vi "tui_ClientSrv Remote File Manager.vi"() -> ()   [LabVIEW 2012]
doc: "Allows management of resource files on the connected server. This makes it feasible to deploy the server in a secure manner while still being able to do some basic maintenance over the network.\n\nNormally, managing files remotely requires you to open a network share. By instead limiting the server's network services to the VI-server protocol, the server becomes less vulnerable. Because all communication goes through one port, it is easy to set up an isolated subnet with forwarding of its VI-server port via an intranet gateway (e.g. using xinetd under linux). That way, the server is accessible from the intranet without being part of it. This is desirable from a security point of view since measurement machines tend to be Windows machines (because of driver support) that must keep on running and thus cannot keep up with the latest security fixes. Such machines should be isolated from the intranet. Indeed, for mission-critical tasks such isolation should be a precondition to deployment no matter how up-to-date the security fixes."
uses:
  served/ClientSrv Server File Manipulation_srv.ctl
  typedefs/t_ClientSrv Remote File Manager States.ctl
  library/typedefs/t_Library Session Methods.ctl
  typedefs/t_ClientSrv Tree Controller Methods.ctl
  typedefs/t_ClientSrv Access Levels.ctl
  typedefs/t_ClientSrv Server File Manipulation Methods.ctl
  library/glb_Library Configuration Globals.vi
panel:
  in  "local start path":path
  in  "remote start path":path
  in  "refresh remote":bool
  in  "delete remote":bool
  in  "rename remote":bool
  in  "mkdir remote":bool
  in  "new remote":bool
  in  "remote tree":string(tree)
  in  "local tree":string(tree)
  in  "refresh local":bool
  in  "delete local":bool
  in  "rename local":bool
  in  "mkdir local":bool
  in  "new local":bool
  out "file manipulation":T1
  in  "pattern":string(combo)
  in  "download":bool
  in  "upload":bool
  in  "exit":bool
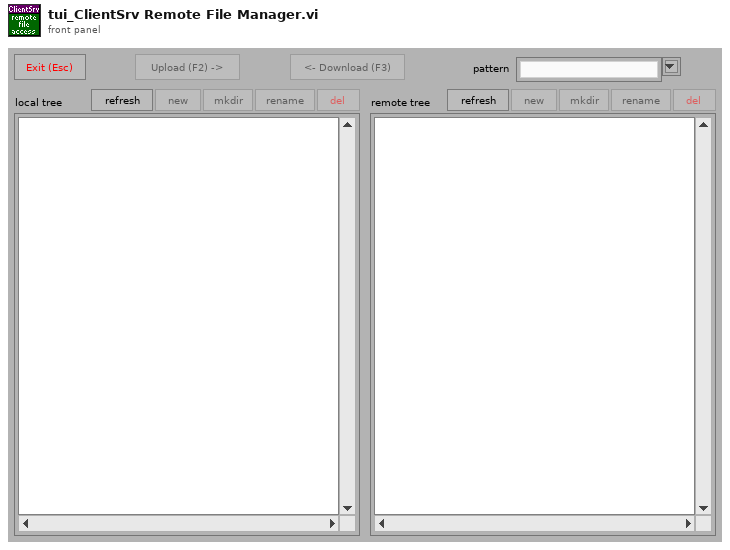
[diagram p1: front panel]
types:
  T1 = typedef "ClientSrv Server File Manipulation_srv.ctl" = refnum<vi>
  T2 = typedef "t_ClientSrv Remote File Manager States.ctl" = enum16{"empty queue", "initialize", "delayed update", "resize", "update trees", "ablement", "cleanup", "stop"}
  T3 = typedef "t_Library Session Methods.ctl" = enum16{"run", "get arg", "set arg", "delist", "cleanup?", "start session", "stop session", "list empty?"}
  T4 = typedef "t_ClientSrv Tree Controller Methods.ctl" = enum16{"do nothing", "initialize", "open item", "close item", "refresh"}
  T5 = typedef "t_ClientSrv Server File Manipulation Methods.ctl" = enum16{"close", "list", "open", "new", "read", "write", "newdir", "info", "rename", "delete"}
  T6 = typedef "t_ClientSrv Access Levels.ctl" = enum16{"observer", "operator", "local"}
  T7 = typedef "eventvkey.ctl" = enum16{"ASCII", "Enter", "Return", "Shift", "Ctrl", "Alt", "Cmd", "Opt", "Caps", "NumLock", "Clear", "Break", "Up", "Down", "Left", "Right", "Insert", "Delete", "Home", "End", "PageUp", "PageDown", "Escape", "Help", "Pause", "ScrollLock", "F1", "F2", "F3", "F4", "F5", "F6", "F7", "F8", "F9", "F10", "F11", "F12", "F13", "F14", "F15", "F16", "F17", "F18", "F19", "F20", "F21", "F22", "F23", "F24", "Play", "VolumeUp", "VolumeDown", "Mute", "Two Byte Char"}
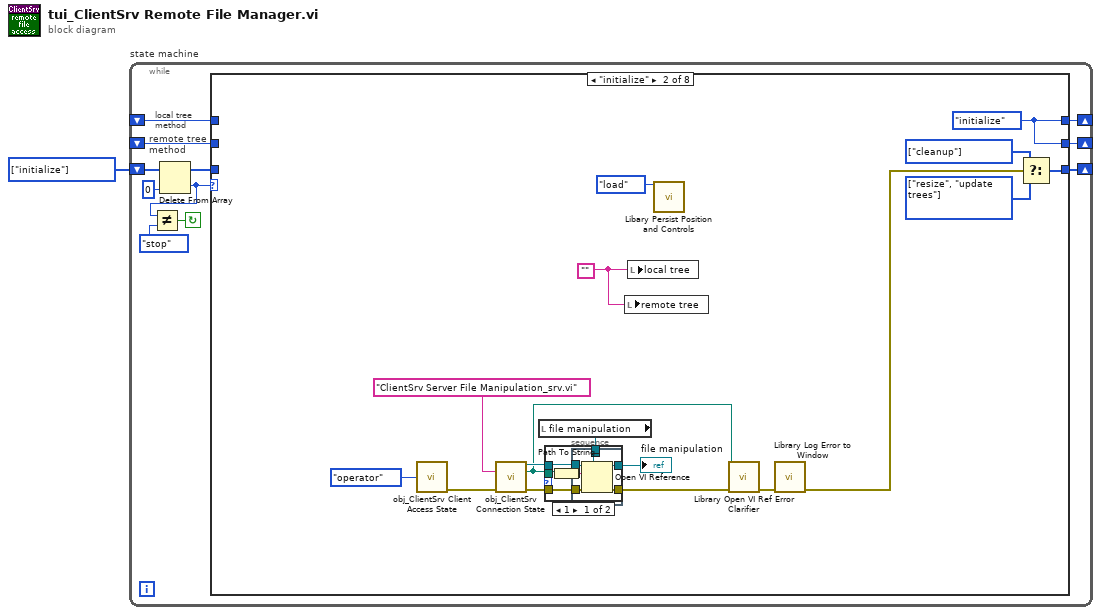
[diagram p0: block diagram]
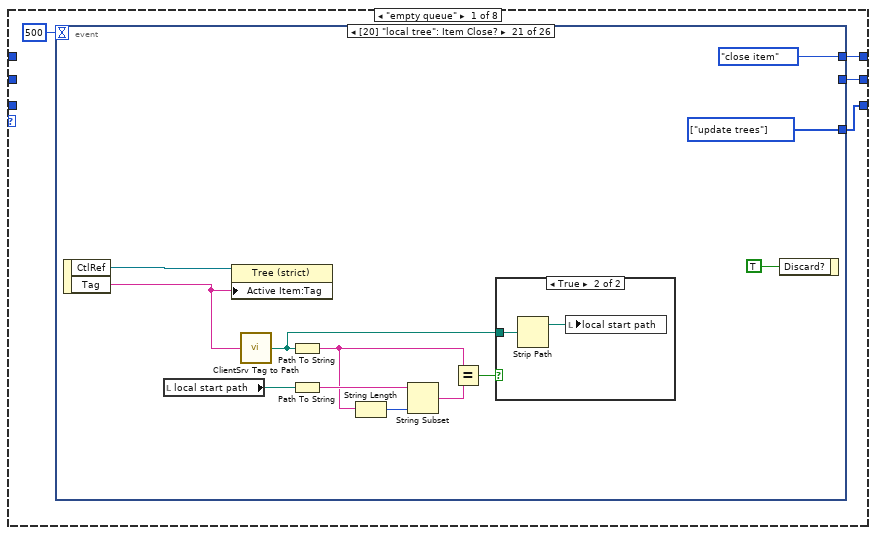
[diagram p2: hidden frame]
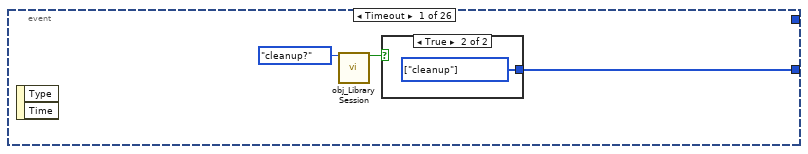
[diagram p3: hidden frame]
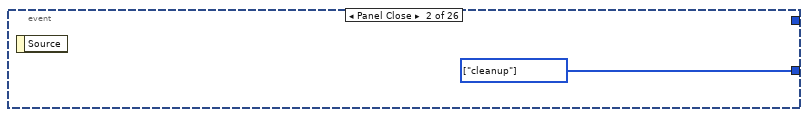
[diagram p5: hidden frame]
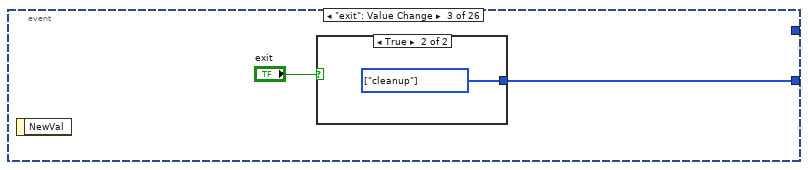
[diagram p6: hidden frame]
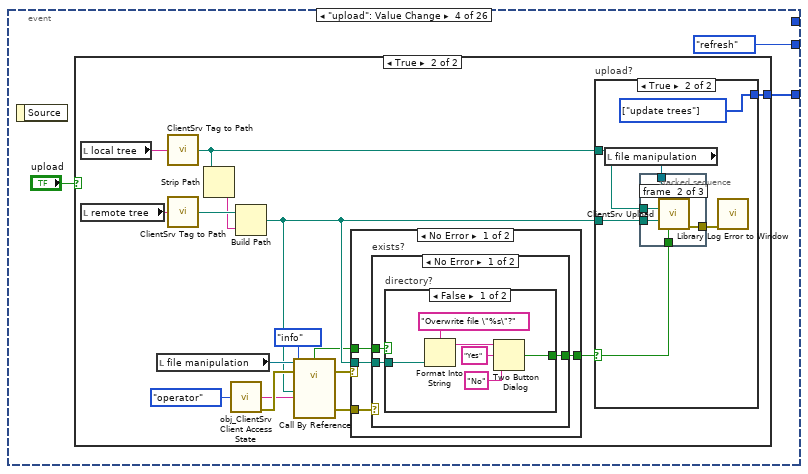
[diagram p8: hidden frame]
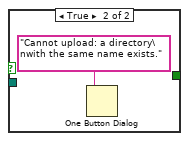
[diagram p10: hidden frame]
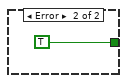
[diagram p11: hidden frame]
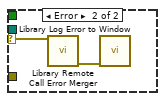
[diagram p12: hidden frame]
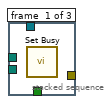
[diagram p14: hidden frame]
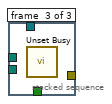
[diagram p15: hidden frame]
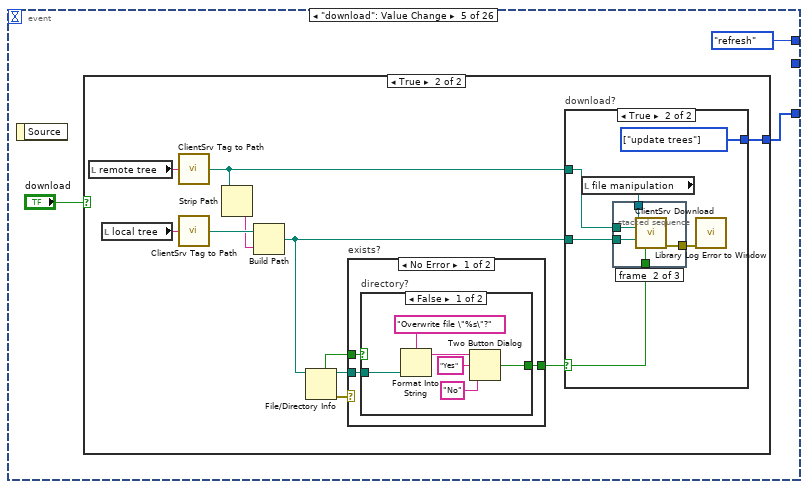
[diagram p16: hidden frame]
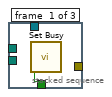
[diagram p19: hidden frame]
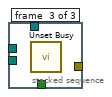
[diagram p20: hidden frame]
diagram:
  w1 = T2[] [enum."initialize"] items=["empty queue", "initialize", "delayed update", "resize", "update trees", "ablement", "cleanup", "stop"]
  n1 = while "state machine" {
    shift-right: [w12] -> _
    shift-left: w1 -> [w5]
    shift-right: [w9] -> _
    shift-left: _ -> [w11]
    shift-right: [w8] -> _
    shift-left: _ -> [w10]
    stop <- w4 continue-if-true
    # "remote tree\nmethod"
    # "local tree\nmethod"
    n2 = Delete From Array(array=w5, index=0) -> (deleted portion=w2:T2, array with subset deleted=w6:T2[])  [unwired: 1 in]
    n3 = Not Equal?(x=w2, y=t_ClientSrv_Remote_File_Manager_States."stop" ("method")) -> (x != y?=w4:bool)
    n4 = case shown="\"initialize\"" w2 {
      tunnel: [w13 w384 w412 w417 w439 w526 w611 w616] -> w12
      tunnel: w6 -> [_ _ w411 w418 w439 w526 _ w616]
      tunnel: w11 -> [_ _ w415 w421 w438 w511 w604 w615]
      tunnel: w10 -> [_ _ w414 w419 w437 w510 w603 w614]
      tunnel: [w15 w388 w415 _ w438 w511 w604 w615] -> w9
      tunnel: [w14 w388 w414 _ w437 w510 w603 w614] -> w8
      frame "empty queue" {
        n5 = event shown="[20] \"local tree\": Item Close?" {
          selector: _ -> [_ _ _ _ _ _ _ _ _ _ _ _ _ _ _ _ _ _ _ _ _ _ _ _ _ _]
          dyn-events: _ -> [_ _ _ _ _ _ _ _ _ _ _ _ _ _ _ _ _ _ _ _ _ _ _ _ _ _]
          timeout: 500 -> [_ _ _ _ _ _ _ _ _ _ _ _ _ _ _ _ _ _ _ _ _ _ _ _ _ _]
          tunnel: [w17 w21 w23 w27 w73 w110 w115 w119 w134 w162 w176 w197 w218 w244 w262 _ _ w320 w326 w340 w354 w358 w360 _ _ w371] -> w13
          tunnel: [_ _ _ t_ClientSrv_Tree_Controller_Methods."refresh" ("Method") _ _ t_ClientSrv_Tree_Controller_Methods."refresh" ("Method") _ w132 _ w174 _ w216 _ w260 _ _ t_ClientSrv_Tree_Controller_Methods."open item" ("Method") _ t_ClientSrv_Tree_Controller_Methods."close item" ("Method") _ _ w359 _ _ _] -> w15
          tunnel: [_ _ _ _ t_ClientSrv_Tree_Controller_Methods."refresh" ("Method") t_ClientSrv_Tree_Controller_Methods."refresh" ("Method") _ w117 _ w161 _ w196 _ w243 _ _ _ _ t_ClientSrv_Tree_Controller_Methods."open item" ("Method") _ t_ClientSrv_Tree_Controller_Methods."close item" ("Method") _ w359 _ _ _] -> w14
          event Timeout {
            n6 = event-data() -> ()  [unwired: 1 in, 2 out]
            n7 = call "obj_Library Session.vi"("method"=t_Library_Session_Methods."cleanup?") -> ("cleanup/empty?"=w18:bool)  [unwired: 11 in, 3 out]
            n8 = case shown="True" w18 {
              tunnel: [_ w20] -> w17
              frame False {
              }
              frame True {
                w20 = T2[] [enum."cleanup"] items=["empty queue", "initialize", "delayed update", "resize", "update trees", "ablement", "cleanup", "stop"]
              }
            }
          }
          event Panel Close {
            w21 = T2[] [enum."cleanup"] items=["empty queue", "initialize", "delayed update", "resize", "update trees", "ablement", "cleanup", "stop"]
            n9 = event-data() -> ()  [unwired: 1 in, 1 out]
          }
          event "exit": Value Change {
            n10 = event-data() -> ()  [unwired: 1 in, 1 out]
            n11 = case shown="True" "exit" {
              tunnel: [_ w24] -> w23
              frame False {
              }
              frame True {
                w24 = T2[] [enum."cleanup"] items=["empty queue", "initialize", "delayed update", "resize", "update trees", "ablement", "cleanup", "stop"]
              }
            }
          }
          event "upload": Value Change {
            n12 = event-data() -> ()  [unwired: 1 in, 1 out]
            n13 = case shown="True" "upload" {
              tunnel: [_ w43] -> w27
              frame False {
              }
              frame True {
                n14 = local read "local tree"() -> (w42:string)
                n15 = local read "remote tree"() -> (w41:string)
                n16 = local read "file manipulation"() -> (w33:T1)
                n17 = call "ClientSrv Tag to Path.vi"("tree tag"=w42) -> ("path"=w37:path)
                n18 = call "ClientSrv Tag to Path.vi"("tree tag"=w41) -> ("path"=w40:path)
                n19 = Strip Path(path=w37) -> (name=w39:string)  [unwired: 1 out]
                n20 = call "obj_ClientSrv Client Access State.vi"("access level (observer)"=t_ClientSrv_Access_Levels."operator") -> ("certificate"=w35:string, "error out"=w36:errorcluster)  [unwired: 13 in]
                n21 = Build Path(base path=w40, name or relative path=w39) -> (appended path=w31:path)
                n22 = call-by-ref "?"(reference=w33, error in=w36, "method"=t_ClientSrv_Server_File_Manipulation_Methods."info", "path"=w31, "certificate"=w35) -> (error out=w28:errorcluster, "directory"=w29:bool, 15:"error out"=w30:errorcluster)  [unwired: 5 in, 7 out]
                n23 = case shown="No Error" w28 {
                  selector: w28 -> [_ w59]
                  tunnel: [w47 _] -> w38
                  tunnel: w31 -> [w46 _]
                  tunnel: w30 -> [w45 _]
                  tunnel: w29 -> [w44 _]
                  frame No Error {
                    n24 = case "exists?" shown="No Error" w45 {
                      tunnel: w44 -> [w50 _]
                      tunnel: w46 -> [w49 _]
                      tunnel: [w48 TRUE ("T button?")] -> w47
                      frame No Error {
                        n25 = case "directory?" shown="False" w50 {
                          tunnel: w49 -> [w55 _]
                          tunnel: [w56 _] -> w48
                          frame False {
                            n26 = Format Into String(format string="Overwrite file \"%s\"?" ("message"), w55) -> (resulting string=w53:string)  [unwired: 2 in, 1 out]
                            n27 = Two Button Dialog(message=w53, 1:"No" ("F button name (\"Cancel\")"), 2:"Yes" ("T button name (\"OK\")")) -> (T button?=w56:bool)
                          }
                          frame True {
                            n28 = One Button Dialog(message="Cannot upload: a directory\nwith the same name exists." ("format string")) -> ()  [unwired: 1 in, 1 out]
                          }
                        }
                      }
                      frame Error {
                      }
                    }
                  }
                  frame Error {
                    n29 = call "Library Remote Call Error Merger.vi"("call by reference node error"=w59) -> ("error out"=w60:errorcluster)  [unwired: 14 in]
                    n30 = call "Library Log Error to Window.vi"("error in (no error)"=w60) -> ()  [unwired: 13 in, 2 out]
                  }
                }
                n31 = case "upload?" shown="True" w38 {
                  selector: w38 -> [_ w65]
                  tunnel: [_ w66] -> w43
                  tunnel: w37 -> [_ w61]
                  tunnel: w31 -> [_ w62]
                  frame False {
                  }
                  frame True {
                    w66 = T2[] [enum."update trees"] items=["empty queue", "initialize", "delayed update", "resize", "update trees", "ablement", "cleanup", "stop"]
                    n32 = local read "file manipulation"() -> (w64:T1)
                    n33 = stacked-sequence {
                      tunnel: w65 -> [_ w71 _]
                      tunnel: w64 -> [_ w70 _]
                      tunnel: [_ w69 _] -> w63
                      tunnel: w62 -> [_ w68 _]
                      tunnel: w61 -> [_ w67 _]
                      frame #0 {
                        n34 = call <vilib>:"Set Busy.vi"() -> ()  [unwired: 10 in, 2 out]
                      }
                      frame #1 {
                        n35 = call "ClientSrv Upload.vi"("file manipulation"=w70, "local file"=w67, "remote file"=w68, "overwrite (F)"=w71) -> ("error out"=w69:errorcluster)  [unwired: 11 in]
                      }
                      frame #2 {
                        n36 = call <vilib>:"Unset Busy.vi"() -> ()  [unwired: 11 in, 1 out]
                      }
                    }
                    n37 = call "Library Log Error to Window.vi"("error in (no error)"=w63) -> ()  [unwired: 13 in, 2 out]
                  }
                }
              }
            }
          }
          event "download": Value Change {
            n38 = event-data() -> ()  [unwired: 1 in, 1 out]
            n39 = case shown="True" "download" {
              tunnel: [_ w85] -> w73
              frame False {
              }
              frame True {
                n40 = local read "remote tree"() -> (w84:string)
                n41 = local read "local tree"() -> (w83:string)
                n42 = call "ClientSrv Tag to Path.vi"("tree tag"=w84) -> ("path"=w76:path)
                n43 = call "ClientSrv Tag to Path.vi"("tree tag"=w83) -> ("path"=w82:path)
                n44 = Strip Path(path=w76) -> (name=w81:string)  [unwired: 1 out]
                n45 = Build Path(base path=w82, name or relative path=w81) -> (appended path=w75:path)
                n46 = File/Directory Info(path=w75) -> (path out=w78:path, directory=w79:bool, error out=w80:errorcluster)  [unwired: 1 in, 4 out]
                n47 = case "exists?" shown="No Error" w80 {
                  tunnel: w79 -> [w100 _]
                  tunnel: w78 -> [w99 _]
                  tunnel: [w98 TRUE ("T button?")] -> w77
                  frame No Error {
                    n48 = case "directory?" shown="False" w100 {
                      tunnel: w99 -> [w105 _]
                      tunnel: [w106 _] -> w98
                      frame False {
                        n49 = Format Into String(format string="Overwrite file \"%s\"?" ("message"), w105) -> (resulting string=w103:string)  [unwired: 2 in, 1 out]
                        n50 = Two Button Dialog(message=w103, 1:"No" ("F button name (\"Cancel\")"), 2:"Yes" ("T button name (\"OK\")")) -> (T button?=w106:bool)
                      }
                      frame True {
                        n51 = One Button Dialog(message="Cannot download: a directory\nwith the same name exists." ("format string")) -> ()  [unwired: 1 in, 1 out]
                      }
                    }
                  }
                  frame Error {
                  }
                }
                n52 = case "download?" shown="True" w77 {
                  selector: w77 -> [_ w90]
                  tunnel: [_ w91] -> w85
                  tunnel: w76 -> [_ w89]
                  tunnel: w75 -> [_ w88]
                  frame False {
                  }
                  frame True {
                    w91 = T2[] [enum."update trees"] items=["empty queue", "initialize", "delayed update", "resize", "update trees", "ablement", "cleanup", "stop"]
                    n53 = local read "file manipulation"() -> (w87:T1)
                    n54 = stacked-sequence {
                      tunnel: w90 -> [w92 w97 _]
                      tunnel: w89 -> [_ w96 _]
                      tunnel: w88 -> [_ w95 _]
                      tunnel: w87 -> [_ w94 _]
                      tunnel: [_ w93 _] -> w86
                      frame #0 {
                        n55 = call <vilib>:"Set Busy.vi"("disable click? (T)"=w92) -> ()  [unwired: 9 in, 2 out]
                      }
                      frame #1 {
                        n56 = call "ClientSrv Download.vi"("file manipulation"=w94, "remote file"=w96, "local file"=w95, "overwrite (F)"=w97) -> ("error out"=w93:errorcluster)  [unwired: 11 in]
                      }
                      frame #2 {
                        n57 = call <vilib>:"Unset Busy.vi"() -> ()  [unwired: 11 in, 1 out]
                      }
                    }
                    n58 = call "Library Log Error to Window.vi"("error in (no error)"=w86) -> ()  [unwired: 13 in, 2 out]
                  }
                }
              }
            }
          }
          event "refresh local": Value Change {
            n59 = event-data() -> ()  [unwired: 1 in, 6 out]
            n60 = case shown="True" "refresh local" {
              tunnel: [_ w112] -> w110
              frame False {
              }
              frame True {
                w112 = T2[] [enum."update trees"] items=["empty queue", "initialize", "delayed update", "resize", "update trees", "ablement", "cleanup", "stop"]
              }
            }
          }
          event "refresh remote": Value Change {
            n61 = event-data() -> ()  [unwired: 1 in, 1 out]
            n62 = case shown="True" "refresh remote" {
              tunnel: [_ w116] -> w115
              frame False {
              }
              frame True {
                w116 = T2[] [enum."update trees"] items=["empty queue", "initialize", "delayed update", "resize", "update trees", "ablement", "cleanup", "stop"]
              }
            }
          }
          event "new local": Value Change {
            n63 = event-data() -> ()  [unwired: 1 in, 1 out]
            n64 = case shown="True" "new local" {
              tunnel: [_ w124] -> w119
              tunnel: [_ t_ClientSrv_Tree_Controller_Methods."refresh" ("Method")] -> w117
              frame False {
              }
              frame True {
                n65 = call "ui_Library Query String.vi"("prompt"="Enter name of new file") -> ("OKed?"=w122:bool, "string out"=w121:string)  [unwired: 13 in]
                n66 = case shown="True" w122 {
                  tunnel: [_ w131] -> w124
                  tunnel: w121 -> [_ w129]
                  frame False {
                  }
                  frame True {
                    w131 = T2[] [enum."update trees"] items=["empty queue", "initialize", "delayed update", "resize", "update trees", "ablement", "cleanup", "stop"]
                    n67 = local read "local tree"() -> (w130:string)
                    n68 = call "ClientSrv Tag to Path.vi"("tree tag"=w130) -> ("path"=w128:path)
                    n69 = Build Path(base path=w128, name or relative path=w129) -> (appended path=w127:path)
                    n70 = call "Library New File.vi"("file path"=w127) -> ("error out"=w126:errorcluster, "refnum"=w125:refnum<file>)  [unwired: 9 in]
                    n71 = Close File(refnum=w125) -> ()  [unwired: 1 in, 2 out]
                    n72 = call "Library Log Error to Window.vi"("error in (no error)"=w126) -> ()  [unwired: 13 in, 2 out]
                  }
                }
              }
            }
          }
          event "new remote": Value Change {
            n73 = event-data() -> ()  [unwired: 1 in, 1 out]
            n74 = case shown="True" "new remote" {
              tunnel: [_ w139] -> w134
              tunnel: [_ t_ClientSrv_Tree_Controller_Methods."refresh" ("Method")] -> w132
              frame False {
              }
              frame True {
                n75 = call "ui_Library Query String.vi"("prompt"="Enter name of new file") -> ("OKed?"=w137:bool, "string out"=w136:string)  [unwired: 13 in]
                n76 = case shown="True" w137 {
                  tunnel: [_ w159] -> w139
                  tunnel: w136 -> [_ w157]
                  frame False {
                  }
                  frame True {
                    w159 = T2[] [enum."update trees"] items=["empty queue", "initialize", "delayed update", "resize", "update trees", "ablement", "cleanup", "stop"]
                    n77 = local read "remote tree"() -> (w158:string)
                    n78 = local read "file manipulation"() -> (w155:T1)
                    n79 = call "ClientSrv Tag to Path.vi"("tree tag"=w158) -> ("path"=w156:path)
                    n80 = call "obj_ClientSrv Client Access State.vi"("access level (observer)"=t_ClientSrv_Access_Levels."operator") -> ("certificate"=w140:string, "error out"=w141:errorcluster)  [unwired: 13 in]
                    n81 = Build Path(base path=w156, name or relative path=w157) -> (appended path=w153:path)
                    n82 = call-by-ref "?"(reference=w155, error in=w141, "method"=t_ClientSrv_Server_File_Manipulation_Methods."new", "path"=w153, "certificate"=w140, "overwrite (F)"=FALSE) -> (reference out=w150:T1, error out=w148:errorcluster, "refnum out"=w149:refnum<file>, 15:"error out"=w147:errorcluster)  [unwired: 4 in, 6 out]
                    n83 = call "Library Remote Call Error Merger.vi"("call by reference node error"=w148, "called VI error (no error)"=w147) -> ("error out"=w146:errorcluster)  [unwired: 13 in]
                    n84 = call-by-ref "?"(reference=w150, error in=w146, "method"=t_ClientSrv_Server_File_Manipulation_Methods."close", "certificate"=w140, "refnum in"=w149) -> (error out=w145:errorcluster, 15:"error out"=w144:errorcluster)  [unwired: 5 in, 8 out]
                    n85 = call "Library Remote Call Error Merger.vi"("call by reference node error"=w145, "called VI error (no error)"=w144) -> ("error out"=w143:errorcluster)  [unwired: 13 in]
                    n86 = call "Library Log Error to Window.vi"("error in (no error)"=w143) -> ()  [unwired: 13 in, 2 out]
                  }
                }
              }
            }
          }
          event "mkdir local": Value Change {
            n87 = event-data() -> ()  [unwired: 1 in, 1 out]
            n88 = case shown="True" "mkdir local" {
              tunnel: [_ w167] -> w162
              tunnel: [_ t_ClientSrv_Tree_Controller_Methods."refresh" ("Method")] -> w161
              frame False {
              }
              frame True {
                n89 = call "ui_Library Query String.vi"("prompt"="Enter name of new directory") -> ("OKed?"=w165:bool, "string out"=w164:string)  [unwired: 13 in]
                n90 = case shown="True" w165 {
                  tunnel: [_ w173] -> w167
                  tunnel: w164 -> [_ w171]
                  frame False {
                  }
                  frame True {
                    w173 = T2[] [enum."delayed update"] items=["empty queue", "initialize", "delayed update", "resize", "update trees", "ablement", "cleanup", "stop"]
                    n91 = local read "local tree"() -> (w172:string)
                    n92 = call "ClientSrv Tag to Path.vi"("tree tag"=w172) -> ("path"=w170:path)
                    n93 = Build Path(base path=w170, name or relative path=w171) -> (appended path=w169:path)
                    n94 = Create Folder(path (use dialog)=w169) -> (error out=w168:errorcluster)  [unwired: 2 in, 2 out]
                    n95 = call "Library Log Error to Window.vi"("error in (no error)"=w168) -> ()  [unwired: 13 in, 2 out]
                  }
                }
              }
            }
          }
          event "mkdir remote": Value Change {
            n96 = event-data() -> ()  [unwired: 1 in, 1 out]
            n97 = case shown="True" "mkdir remote" {
              tunnel: [_ w181] -> w176
              tunnel: [_ t_ClientSrv_Tree_Controller_Methods."refresh" ("Method")] -> w174
              frame False {
              }
              frame True {
                n98 = call "ui_Library Query String.vi"("prompt"="Enter name of new directory") -> ("OKed?"=w179:bool, "string out"=w178:string)  [unwired: 13 in]
                n99 = case shown="True" w179 {
                  tunnel: [_ w194] -> w181
                  tunnel: w178 -> [_ w192]
                  frame False {
                  }
                  frame True {
                    w194 = T2[] [enum."delayed update"] items=["empty queue", "initialize", "delayed update", "resize", "update trees", "ablement", "cleanup", "stop"]
                    n100 = local read "remote tree"() -> (w193:string)
                    n101 = call "ClientSrv Tag to Path.vi"("tree tag"=w193) -> ("path"=w191:path)
                    n102 = local read "file manipulation"() -> (w190:T1)
                    n103 = Build Path(base path=w191, name or relative path=w192) -> (appended path=w184:path)
                    n104 = call "obj_ClientSrv Client Access State.vi"("access level (observer)"=t_ClientSrv_Access_Levels."operator") -> ("certificate"=w185:string, "error out"=w182:errorcluster)  [unwired: 13 in]
                    n105 = call-by-ref "?"(reference=w190, error in=w182, "method"=t_ClientSrv_Server_File_Manipulation_Methods."newdir", "path"=w184, "certificate"=w185) -> (error out=w188:errorcluster, 15:"error out"=w187:errorcluster)  [unwired: 5 in, 8 out]
                    n106 = call "Library Remote Call Error Merger.vi"("call by reference node error"=w188, "called VI error (no error)"=w187) -> ("error out"=w183:errorcluster)  [unwired: 13 in]
                    n107 = call "Library Log Error to Window.vi"("error in (no error)"=w183) -> ()  [unwired: 13 in, 2 out]
                  }
                }
              }
            }
          }
          event "rename local": Value Change {
            n108 = event-data() -> ()  [unwired: 1 in, 1 out]
            n109 = case shown="True" "rename local" {
              tunnel: [_ w209] -> w197
              tunnel: [_ t_ClientSrv_Tree_Controller_Methods."refresh" ("Method")] -> w196
              frame False {
              }
              frame True {
                n110 = local read "local tree"() -> (w207:string)
                n111 = call "ClientSrv Tag to Path.vi"("tree tag"=w207) -> ("path"=w205:path)
                n112 = Strip Path(path=w205) -> (stripped path=w206:path, name=w203:string)
                n113 = call "ui_Library Query String.vi"("prompt"="Specify a new name", "string in (\"\")"=w203) -> ("OKed?"=w201:bool, "string out"=w199:string)  [unwired: 12 in]
                n114 = Not Equal?(x=w203, y=w199) -> (x != y?=w200:bool)
                n115 = Empty String/Path?(string/path=w199) -> (empty?=w198:bool)
                n116 = Compound Arithmetic op=AND(w200, w201, invert w198) -> (w202:bool)
                n117 = case "name OKed and different and not empty?" shown="True" w202 {
                  tunnel: [_ w215] -> w209
                  tunnel: w206 -> [_ w213]
                  tunnel: w199 -> [_ w212]
                  tunnel: w205 -> [_ w210]
                  frame False {
                  }
                  frame True {
                    w215 = T2[] [enum."delayed update"] items=["empty queue", "initialize", "delayed update", "resize", "update trees", "ablement", "cleanup", "stop"]
                    n118 = Build Path(base path=w213, name or relative path=w212) -> (appended path=w211:path)
                    n119 = Move(source path=w210, 10:w211) -> (error out=w214:errorcluster)  [unwired: 3 in, 2 out]
                    n120 = call "Library Log Error to Window.vi"("error in (no error)"=w214) -> ()  [unwired: 13 in, 2 out]
                  }
                }
              }
            }
          }
          event "rename remote": Value Change {
            n121 = event-data() -> ()  [unwired: 1 in, 1 out]
            n122 = case shown="True" "rename remote" {
              tunnel: [_ w230] -> w218
              tunnel: [_ t_ClientSrv_Tree_Controller_Methods."refresh" ("Method")] -> w216
              frame False {
              }
              frame True {
                n123 = local read "remote tree"() -> (w229:string)
                n124 = call "ClientSrv Tag to Path.vi"("tree tag"=w229) -> ("path"=w227:path)
                n125 = Strip Path(path=w227) -> (stripped path=w228:path, name=w225:string)
                n126 = call "ui_Library Query String.vi"("prompt"="Specify a new name", "string in (\"\")"=w225) -> ("OKed?"=w223:bool, "string out"=w221:string)  [unwired: 12 in]
                n127 = Not Equal?(x=w225, y=w221) -> (x != y?=w222:bool)
                n128 = Empty String/Path?(string/path=w221) -> (empty?=w220:bool)
                n129 = Compound Arithmetic op=AND(w222, w223, invert w220) -> (w224:bool)
                n130 = case "name OKed and different and not empty?" shown="True" w224 {
                  tunnel: [_ w241] -> w230
                  tunnel: w228 -> [_ _]
                  tunnel: w221 -> [_ w231]
                  tunnel: w227 -> [_ w232]
                  frame False {
                  }
                  frame True {
                    w241 = T2[] [enum."delayed update"] items=["empty queue", "initialize", "delayed update", "resize", "update trees", "ablement", "cleanup", "stop"]
                    n131 = local read "file manipulation"() -> (w240:T1)
                    n132 = call "obj_ClientSrv Client Access State.vi"("access level (observer)"=t_ClientSrv_Access_Levels."operator") -> ("certificate"=w235:string, "error out"=w233:errorcluster)  [unwired: 13 in]
                    n133 = call-by-ref "?"(reference=w240, error in=w233, "method"=t_ClientSrv_Server_File_Manipulation_Methods."rename", "new name"=w231, "path"=w232, "certificate"=w235) -> (error out=w238:errorcluster, 15:"error out"=w237:errorcluster)  [unwired: 4 in, 8 out]
                    n134 = call "Library Remote Call Error Merger.vi"("call by reference node error"=w238, "called VI error (no error)"=w237) -> ("error out"=w234:errorcluster)  [unwired: 13 in]
                    n135 = call "Library Log Error to Window.vi"("error in (no error)"=w234) -> ()  [unwired: 13 in, 2 out]
                  }
                }
              }
            }
          }
          event "delete local": Value Change {
            n136 = event-data() -> ()  [unwired: 1 in, 1 out]
            n137 = case shown="True" "delete local" {
              tunnel: [_ w256] -> w244
              tunnel: [_ t_ClientSrv_Tree_Controller_Methods."refresh" ("Method")] -> w243
              frame False {
              }
              frame True {
                n138 = local read "local tree"() -> (w253:string)
                n139 = call "ClientSrv Tag to Path.vi"("tree tag"=w253) -> ("path"=w254:path)
                n140 = property on="local tree" class="Tree (strict)"("Active Item:Tag"=w253) -> ("Active Item:Child-Only?"=w252:bool)  [unwired: 2 in, 2 out]
                n141 = Select(t="file", s=w252, f="directory") -> (s? t:f=w248:string)
                n142 = Strip Path(path=w254) -> (name=w249:string)  [unwired: 1 out]
                n143 = Format Into String(format string="Delete %s \"%s\"?", w248, w249) -> (resulting string=w246:string)  [unwired: 2 in, 1 out]
                n144 = Two Button Dialog(message=w246) -> (T button?=w245:bool)  [unwired: 2 in]
                n145 = case "OK?" shown="True" w245 {
                  tunnel: [_ w259] -> w256
                  tunnel: w254 -> [_ w258]
                  frame False {
                  }
                  frame True {
                    w259 = T2[] [enum."delayed update"] items=["empty queue", "initialize", "delayed update", "resize", "update trees", "ablement", "cleanup", "stop"]
                    n146 = Delete(path (use dialog)=w258) -> (error out=w257:errorcluster)  [unwired: 4 in, 2 out]
                    n147 = call "Library Log Error to Window.vi"("error in (no error)"=w257) -> ()  [unwired: 13 in, 2 out]
                  }
                }
              }
            }
          }
          event "delete remote": Value Change {
            n148 = event-data() -> ()  [unwired: 1 in, 1 out]
            n149 = case shown="True" "delete remote" {
              tunnel: [_ w274] -> w262
              tunnel: [_ t_ClientSrv_Tree_Controller_Methods."refresh" ("Method")] -> w260
              frame False {
              }
              frame True {
                n150 = local read "remote tree"() -> (w272:string)
                n151 = property on="remote tree" class="Tree (strict)"("Active Item:Tag"=w272) -> ("Active Item:Child-Only?"=w271:bool)  [unwired: 2 in, 2 out]
                n152 = call "ClientSrv Tag to Path.vi"("tree tag"=w272) -> ("path"=w273:path)
                n153 = Select(t="file", s=w271, f="directory") -> (s? t:f=w267:string)
                n154 = Strip Path(path=w273) -> (name=w268:string)  [unwired: 1 out]
                n155 = Format Into String(format string="Delete %s \"%s\"?", w267, w268) -> (resulting string=w265:string)  [unwired: 2 in, 1 out]
                n156 = Two Button Dialog(message=w265) -> (T button?=w264:bool)  [unwired: 2 in]
                n157 = case "OK?" shown="True" w264 {
                  tunnel: [_ w284] -> w274
                  tunnel: w273 -> [_ w275]
                  frame False {
                  }
                  frame True {
                    w284 = T2[] [enum."delayed update"] items=["empty queue", "initialize", "delayed update", "resize", "update trees", "ablement", "cleanup", "stop"]
                    n158 = local read "file manipulation"() -> (w276:T1)
                    n159 = call "obj_ClientSrv Client Access State.vi"("access level (observer)"=t_ClientSrv_Access_Levels."operator") -> ("certificate"=w281:string, "error out"=w283:errorcluster)  [unwired: 13 in]
                    n160 = call-by-ref "?"(reference=w276, error in=w283, "method"=t_ClientSrv_Server_File_Manipulation_Methods."delete", "path"=w275, "certificate"=w281) -> (error out=w278:errorcluster, 15:"error out"=w279:errorcluster)  [unwired: 5 in, 8 out]
                    n161 = call "Library Remote Call Error Merger.vi"("call by reference node error"=w278, "called VI error (no error)"=w279) -> ("error out"=w282:errorcluster)  [unwired: 13 in]
                    n162 = call "Library Log Error to Window.vi"("error in (no error)"=w282) -> ()  [unwired: 13 in, 2 out]
                  }
                }
              }
            }
          }
          event "local tree": Double Click {
            n163 = event-data() -> ("CtlRef"=w288:refnum<vi>)  [unwired: 1 in]
            n164 = invoke class="Tree (strict)" method="Double Click"(reference=w288) -> (reference out=w287:refnum<vi>, "Double Click"=w286:string)  [unwired: 2 in, 1 out]
            n165 = property class="Tree (strict)"(reference=w287, "Active Item:Tag"=w286) -> ("Active Item:Child-Only?"=w285:bool)  [unwired: 1 in, 2 out]
            n166 = case shown="True" w285 {
              tunnel: w286 -> [_ w297]
              frame False {
              }
              frame True {
                n167 = call "ClientSrv Tag to Path.vi"("tree tag"=w297) -> ("path"=w296:path)
                n168 = File/Directory Info(path=w296) -> (size=w289:i64, last mod=w293:timestamp)  [unwired: 1 in, 5 out]
                n169 = To Long Integer(number=w289) -> (32bit integer=w295:i32)
                n170 = global read "glb_Library Configuration Globals.vi" "time format"() -> (w294:string)
                n171 = Format Date/Time String(time format string (%c)=w294, seconds (now)=w293) -> (date/time string=w292:string)  [unwired: 1 in]
                n172 = Format Into String(format string="Size: %d bytes.\nLast modified: %s", w295, w292) -> (resulting string=w290:string)  [unwired: 2 in, 1 out]
                n173 = One Button Dialog(message=w290) -> ()  [unwired: 1 in, 1 out]
              }
            }
          }
          event "remote tree": Double Click {
            n174 = event-data() -> ("CtlRef"=w301:refnum<vi>)  [unwired: 1 in]
            n175 = invoke class="Tree (strict)" method="Double Click"(reference=w301) -> (reference out=w300:refnum<vi>, "Double Click"=w299:string)  [unwired: 2 in, 1 out]
            n176 = property class="Tree (strict)"(reference=w300, "Active Item:Tag"=w299) -> ("Active Item:Child-Only?"=w298:bool)  [unwired: 1 in, 2 out]
            n177 = case shown="True" w298 {
              tunnel: w299 -> [_ w317]
              frame False {
              }
              frame True {
                n178 = local read "file manipulation"() -> (w305:T1)
                n179 = call "ClientSrv Tag to Path.vi"("tree tag"=w317) -> ("path"=w304:path)
                n180 = call "obj_ClientSrv Client Access State.vi"("access level (observer)"=t_ClientSrv_Access_Levels."operator") -> ("certificate"=w310:string, "error out"=w312:errorcluster)  [unwired: 13 in]
                n181 = call-by-ref "?"(reference=w305, error in=w312, "method"=t_ClientSrv_Server_File_Manipulation_Methods."info", "path"=w304, "certificate"=w310) -> (error out=w307:errorcluster, "last mod"=w302:timestamp, "length"=w303:i32, 15:"error out"=w308:errorcluster)  [unwired: 5 in, 6 out]
                n182 = call "Library Remote Call Error Merger.vi"("call by reference node error"=w307, "called VI error (no error)"=w308) -> ("error out"=w311:errorcluster)  [unwired: 13 in]
                n183 = global read "glb_Library Configuration Globals.vi" "time format"() -> (w316:string)
                n184 = call "Library Log Error to Window.vi"("error in (no error)"=w311) -> ()  [unwired: 13 in, 2 out]
                n185 = Format Date/Time String(time format string (%c)=w316, seconds (now)=w302) -> (date/time string=w315:string)  [unwired: 1 in]
                n186 = Format Into String(format string="Size: %d bytes.\nLast modified: %s", w303, w315) -> (resulting string=w313:string)  [unwired: 2 in, 1 out]
                n187 = One Button Dialog(message=w313) -> ()  [unwired: 1 in, 1 out]
              }
            }
          }
          event "remote tree": Item Open? {
            w320 = T2[] [enum."update trees"] items=["empty queue", "initialize", "delayed update", "resize", "update trees", "ablement", "cleanup", "stop"]
            n188 = event-data() -> ("CtlRef"=w321:refnum<vi>, "Tag"=w318:string)  [unwired: 1 in]
            n189 = property class="Tree (strict)"(reference=w321, "Active Item:Tag"=w318) -> ()  [unwired: 1 in, 2 out]
            n190 = call "ClientSrv Tag to Path.vi"("tree tag"=w318) -> ("path"=w319:path)
            n191 = local write "remote start path"(w319) -> ()
            n192 = event-data("Discard?"=TRUE) -> ()  [unwired: 1 in, 1 out]
          }
          event "local tree": Item Open? {
            w326 = T2[] [enum."update trees"] items=["empty queue", "initialize", "delayed update", "resize", "update trees", "ablement", "cleanup", "stop"]
            n193 = event-data() -> ("CtlRef"=w327:refnum<vi>, "Tag"=w325:string)  [unwired: 1 in]
            n194 = property class="Tree (strict)"(reference=w327, "Active Item:Tag"=w325) -> ()  [unwired: 1 in, 2 out]
            n195 = call "ClientSrv Tag to Path.vi"("tree tag"=w325) -> ("path"=w324:path)
            n196 = local write "local start path"(w324) -> ()
            n197 = event-data("Discard?"=TRUE) -> ()  [unwired: 1 in, 1 out]
          }
          event "remote tree": event type 3.0.x80000011 {
            w340 = T2[] [enum."update trees"] items=["empty queue", "initialize", "delayed update", "resize", "update trees", "ablement", "cleanup", "stop"]
            n198 = event-data() -> ("CtlRef"=w336:refnum<vi>, "Tag"=w335:string)  [unwired: 1 in]
            n199 = local read "remote start path"() -> (w338:path)
            n200 = property class="Tree (strict)"(reference=w336, "Active Item:Tag"=w335) -> ()  [unwired: 1 in, 2 out]
            n201 = call "ClientSrv Tag to Path.vi"("tree tag"=w335) -> ("path"=w330:path)
            n202 = Path To String(path=w330) -> (string=w331:string)
            n203 = Path To String(path=w338) -> (string=w334:string)
            n204 = String Length(string=w331) -> (length=w332:i32)
            n205 = String Subset(string=w334, length (rest)=w332) -> (substring=w333:string)  [unwired: 1 in]
            n206 = Equal?(x=w331, y=w333) -> (x = y?=w337:bool)
            n207 = case shown="True" w337 {
              tunnel: w330 -> [_ w342]
              frame False {
              }
              frame True {
                n208 = Strip Path(path=w342) -> (stripped path=w343:path)  [unwired: 1 out]
                n209 = local write "remote start path"(w343) -> ()
              }
            }
            n210 = event-data("Discard?"=TRUE) -> ()  [unwired: 1 in, 1 out]
          }
          event "local tree": event type 3.0.x80000011 {
            w354 = T2[] [enum."update trees"] items=["empty queue", "initialize", "delayed update", "resize", "update trees", "ablement", "cleanup", "stop"]
            n211 = event-data() -> ("CtlRef"=w345:refnum<vi>, "Tag"=w344:string)  [unwired: 1 in]
            n212 = local read "local start path"() -> (w352:path)
            n213 = property class="Tree (strict)"(reference=w345, "Active Item:Tag"=w344) -> ()  [unwired: 1 in, 2 out]
            n214 = call "ClientSrv Tag to Path.vi"("tree tag"=w344) -> ("path"=w346:path)
            n215 = Path To String(path=w346) -> (string=w347:string)
            n216 = Path To String(path=w352) -> (string=w350:string)
            n217 = String Length(string=w347) -> (length=w348:i32)
            n218 = String Subset(string=w350, length (rest)=w348) -> (substring=w349:string)  [unwired: 1 in]
            n219 = Equal?(x=w347, y=w349) -> (x = y?=w351:bool)
            n220 = case shown="True" w351 {
              tunnel: w346 -> [_ w356]
              frame False {
              }
              frame True {
                n221 = Strip Path(path=w356) -> (stripped path=w357:path)  [unwired: 1 out]
                n222 = local write "local start path"(w357) -> ()
              }
            }
            n223 = event-data("Discard?"=TRUE) -> ()  [unwired: 1 in, 1 out]
          }
          event "local tree", "remote tree": Value Change {
            w358 = T2[] [enum."ablement"] items=["empty queue", "initialize", "delayed update", "resize", "update trees", "ablement", "cleanup", "stop"]
            n224 = event-data() -> ()  [unwired: 1 in, 1 out]
          }
          event "pattern": Value Change {
            w360 = T2[] [enum."update trees"] items=["empty queue", "initialize", "delayed update", "resize", "update trees", "ablement", "cleanup", "stop"]
            w359 = t_ClientSrv_Tree_Controller_Methods."refresh" ("Method")
            n225 = event-data() -> ()  [unwired: 1 in, 1 out]
          }
          event Key Down? {
            n226 = event-data() -> ("VKey"=w361:T7)  [unwired: 1 in]
            n227 = call <vilib>:"compatReturnToEnter.vi"("VKey"=w361) -> ("VKey"=w363:T7)
            n228 = case shown="\"F1\"" w363 {
              tunnel: [FALSE TRUE] -> w362
              frame Default {
              }
              frame "F1" {
                n229 = call "Library Show Help.vi"() -> ()  [unwired: 1 in]
              }
            }
            n230 = event-data("Discard?"=w362) -> ()  [unwired: 1 in, 1 out]
          }
          event event type 5.0.x8000000b {
            n231 = event-data() -> ("VKey"=w366:T7)  [unwired: 1 in]
            n232 = call <vilib>:"compatReturnToEnter.vi"("VKey"=w366) -> ("VKey"=w368:T7)
            n233 = case shown="\"F1\"" w368 {
              tunnel: [FALSE TRUE] -> w367
              frame Default {
              }
              frame "F1" {
              }
            }
            n234 = event-data("Discard?"=w367) -> ()  [unwired: 1 in, 1 out]
          }
          event Panel Resize {
            w371 = T2[] [enum."resize"] items=["empty queue", "initialize", "delayed update", "resize", "update trees", "ablement", "cleanup", "stop"]
            n235 = event-data() -> ()  [unwired: 1 in, 1 out]
          }
        }
      }
      frame "initialize" {
        w381 = T2[] [enum."cleanup"] items=["empty queue", "initialize", "delayed update", "resize", "update trees", "ablement", "cleanup", "stop"]
        w387 = ""
        w388 = t_ClientSrv_Tree_Controller_Methods."initialize" ("Method")
        w383 = T2[] [enum."resize", enum."update trees"] items=["empty queue", "initialize", "delayed update", "resize", "update trees", "ablement", "cleanup", "stop"]
        n236 = call "obj_ClientSrv Client Access State.vi"("access level (observer)"=t_ClientSrv_Access_Levels."operator") -> ("error out"=w379:errorcluster)  [unwired: 13 in, 1 out]
        n237 = call "obj_ClientSrv Connection State.vi"("machine{connect}/VI{get state} name (local/no path resolution)"="ClientSrv Server File Manipulation_srv.vi", "error in (no error)"=w379) -> ("server app ref"=w375:refnum<vi>, "resolved server path"=w374:path, "error out"=w376:errorcluster)  [unwired: 6 in, 5 out]
        n238 = local read "file manipulation"() -> (w372:T1)
        n239 = stacked-sequence {
          tunnel: [w394] -> w373
          tunnel: [w393] -> w377
          tunnel: w376 -> [w392]
          tunnel: w375 -> [w391]
          tunnel: w374 -> [w390]
          tunnel: w372 -> [w389]
          frame #0 {
            # "avoid LV8 complaints"
            n240 = Path to Array of Strings(0:w390) -> (2:w395:string[])  [unwired: 1 out]
            n241 = Array Size(array=w395) -> (size(s)=w396:i32)
            n242 = case shown="1" w396 {
              tunnel: w390 -> [w403 w409]
              tunnel: w391 -> [w401 w408]
              tunnel: [w399 w404] -> w394
              tunnel: [w397 w407] -> w393
              tunnel: w389 -> [w398 w406]
              tunnel: w392 -> [w400 w405]
              frame 1 {
                n243 = Path To String(path=w403) -> (string=w402:string)
                n244 = Open VI Reference(type specifier VI Refnum (for type only)=w398, application reference (local)=w401, vi path=w402, error in (no error)=w400) -> (vi reference=w399:T1, error out=w397:errorcluster)  [unwired: 2 in]
              }
              frame Default {
                n245 = Open VI Reference(type specifier VI Refnum (for type only)=w406, application reference (local)=w408, vi path=w409, error in (no error)=w405) -> (vi reference=w404:T1, error out=w407:errorcluster)  [unwired: 2 in]
              }
            }
          }
        }
        "file manipulation" <- w373
        n246 = local write "remote tree"(w387) -> ()
        n247 = local write "local tree"(w387) -> ()
        n248 = call "Libary Persist Position and Controls.vi"("action"=enum16{"save", "load"}."load") -> ()  [unwired: 13 in, 2 out]
        n249 = call "Library Open VI Ref Error Clarifier.vi"("VI path"=w374, "called VI error (no error)"=w377) -> ("error out"=w385:errorcluster)  [unwired: 13 in]
        n250 = call "Library Log Error to Window.vi"("error in (no error)"=w385) -> ("dup error"=w382:errorcluster)  [unwired: 13 in, 1 out]
        n251 = Select(t=w381, s=w382, f=w383) -> (s? t:f=w384:T2[])
      }
      frame "delayed update" {
        # "Some file I/O operations seem to take a\nwhile before they register. To prevent\nthe old state from being displayed when\nupdating the tree, it can be scheduled\nvia this state to insert a small wait."
        n252 = Wait (ms)(milliseconds to wait=u32 50) -> ()  [unwired: 1 out]
        n253 = Build Array (concatenate)(t_ClientSrv_Remote_File_Manager_States."update trees" ("method"), w411) -> (w412:T2[])
      }
      frame "update trees" {
        n254 = flat-sequence {
          tunnel: [w426] -> w422
          tunnel: w421 -> [w426]
          tunnel: [w425] -> w420
          tunnel: w419 -> [w425]
          tunnel: w422 -> [w434]
          tunnel: w420 -> [w433]
          frame #0 {
            n255 = property class="VI"() -> ("Front Panel"=w423:refnum<vi>)  [unwired: 2 in, 2 out]
            n256 = call <vilib>:"Set Busy.vi"() -> ()  [unwired: 10 in, 2 out]
            n257 = property class="Pnl"(reference=w423, "Defer Panel Updates"=TRUE) -> ()  [unwired: 1 in, 2 out]
          }
          frame #1 {
            n258 = local read "file manipulation"() -> (w432:T1)
            n259 = control-ref of="local tree"() -> (w429:refnum<vi>)
            n260 = control-ref of="remote tree"() -> (w430:refnum<vi>)
            n261 = call "re_ClientSrv Tree Controller.vi"("method"=w433, "start path"="local start path", "tree control reference"=w429, "pattern"="pattern") -> ()  [unwired: 12 in]
            n262 = call "re_ClientSrv Tree Controller.vi"("method"=w434, "start path"="remote start path", "tree control reference"=w430, "pattern"="pattern", "file manipulation (local)"=w432) -> ()  [unwired: 11 in]
          }
          frame #2 {
            n263 = property class="VI"() -> ("Front Panel"=w436:refnum<vi>)  [unwired: 2 in, 2 out]
            n264 = call <vilib>:"Unset Busy.vi"() -> ()  [unwired: 11 in, 1 out]
            n265 = property class="Pnl"(reference=w436, "Defer Panel Updates"=FALSE) -> ()  [unwired: 1 in, 2 out]
          }
        }
        n266 = Build Array (concatenate)(t_ClientSrv_Remote_File_Manager_States."ablement" ("method"), w418) -> (w417:T2[])
      }
      frame "resize" {
        n267 = flat-sequence {
          frame #0 {
            n268 = property class="VI"() -> ("Front Panel"=w440:refnum<vi>)  [unwired: 2 in, 2 out]
            n269 = property class="Pnl"(reference=w440, "Defer Panel Updates"=TRUE) -> ()  [unwired: 1 in, 2 out]
          }
          frame #1 {
            n270 = property on="local tree" class="Tree (strict)"() -> ("Position:Top"=w465:i32, "Position:Left"=w462:i32, "Bounds:Width"=w461:u32)  [unwired: 2 in, 2 out]
            n271 = property on="delete local" class="Bool"() -> ("Position:Left"=w451:i32, "Bounds:Width"=w450:u32)  [unwired: 2 in, 2 out]
            n272 = property on="remote tree" class="Tree (strict)"() -> ("Position:Top"=w455:i32, "Position:Left"=w457:i32, "Bounds:Width"=w458:u32)  [unwired: 2 in, 2 out]
            n273 = property on="delete remote" class="Bool"() -> ("Position:Left"=w452:i32, "Bounds:Width"=w453:u32)  [unwired: 2 in, 2 out]
            n274 = To Long Integer(number=w461) -> (32bit integer=w460:i32)
            n275 = To Long Integer(number=w450) -> (32bit integer=w449:i32)
            n276 = To Long Integer(number=w458) -> (32bit integer=w459:i32)
            n277 = To Long Integer(number=w453) -> (32bit integer=w454:i32)
            n278 = Add(x=w462, y=w460) -> (x+y=w448:i32)
            n279 = Add(x=w451, y=w449) -> (x+y=w447:i32)
            n280 = Add(x=w457, y=w459) -> (x+y=w443:i32)
            n281 = Add(x=w452, y=w454) -> (x+y=w442:i32)
            n282 = Subtract(x=w465, y=7) -> (x-y=w463:i32)
            n283 = Subtract(x=w455, y=7) -> (x-y=w445:i32)
            n284 = Subtract(x=w448, y=w447) -> (x-y=w446:i32)
            n285 = Subtract(x=w443, y=w442) -> (x-y=w444:i32)
            n286 = stacked-sequence {
              tunnel: w463 -> [w489 w493 w497 w501 w505]
              tunnel: w446 -> [w486 w490 w494 w498 w502]
              frame #0 {
                n287 = property on="refresh local" class="Bool"() -> ("Position:Left"=w488:i32)  [unwired: 2 in, 2 out]
                n288 = Add(x=w488, y=w486) -> (x+y=w487:i32)
                n289 = property on="refresh local" class="Bool"("Position:Top"=w489, "Position:Left"=w487) -> ()  [unwired: 2 in, 2 out]
              }
              frame #1 {
                n290 = property on="delete local" class="Bool"() -> ("Position:Left"=w492:i32)  [unwired: 2 in, 2 out]
                n291 = Add(x=w492, y=w490) -> (x+y=w491:i32)
                n292 = property on="delete local" class="Bool"("Position:Top"=w493, "Position:Left"=w491) -> ()  [unwired: 2 in, 2 out]
              }
              frame #2 {
                n293 = property on="rename local" class="Bool"() -> ("Position:Left"=w496:i32)  [unwired: 2 in, 2 out]
                n294 = Add(x=w496, y=w494) -> (x+y=w495:i32)
                n295 = property on="rename local" class="Bool"("Position:Top"=w497, "Position:Left"=w495) -> ()  [unwired: 2 in, 2 out]
              }
              frame #3 {
                n296 = property on="mkdir local" class="Bool"() -> ("Position:Left"=w500:i32)  [unwired: 2 in, 2 out]
                n297 = Add(x=w500, y=w498) -> (x+y=w499:i32)
                n298 = property on="mkdir local" class="Bool"("Position:Top"=w501, "Position:Left"=w499) -> ()  [unwired: 2 in, 2 out]
              }
              frame #4 {
                n299 = property on="new local" class="Bool"() -> ("Position:Left"=w504:i32)  [unwired: 2 in, 2 out]
                n300 = Add(x=w504, y=w502) -> (x+y=w503:i32)
                n301 = property on="new local" class="Bool"("Position:Top"=w505, "Position:Left"=w503) -> ()  [unwired: 2 in, 2 out]
              }
            }
            n302 = stacked-sequence {
              tunnel: w445 -> [w469 w473 w477 w481 w485]
              tunnel: w444 -> [w466 w470 w474 w478 w482]
              frame #0 {
                n303 = property on="refresh remote" class="Bool"() -> ("Position:Left"=w468:i32)  [unwired: 2 in, 2 out]
                n304 = Add(x=w468, y=w466) -> (x+y=w467:i32)
                n305 = property on="refresh remote" class="Bool"("Position:Top"=w469, "Position:Left"=w467) -> ()  [unwired: 2 in, 2 out]
              }
              frame #1 {
                n306 = property on="delete remote" class="Bool"() -> ("Position:Left"=w472:i32)  [unwired: 2 in, 2 out]
                n307 = Add(x=w472, y=w470) -> (x+y=w471:i32)
                n308 = property on="delete remote" class="Bool"("Position:Top"=w473, "Position:Left"=w471) -> ()  [unwired: 2 in, 2 out]
              }
              frame #2 {
                n309 = property on="rename remote" class="Bool"() -> ("Position:Left"=w476:i32)  [unwired: 2 in, 2 out]
                n310 = Add(x=w476, y=w474) -> (x+y=w475:i32)
                n311 = property on="rename remote" class="Bool"("Position:Top"=w477, "Position:Left"=w475) -> ()  [unwired: 2 in, 2 out]
              }
              frame #3 {
                n312 = property on="mkdir remote" class="Bool"() -> ("Position:Left"=w480:i32)  [unwired: 2 in, 2 out]
                n313 = Add(x=w480, y=w478) -> (x+y=w479:i32)
                n314 = property on="mkdir remote" class="Bool"("Position:Top"=w481, "Position:Left"=w479) -> ()  [unwired: 2 in, 2 out]
              }
              frame #4 {
                n315 = property on="new remote" class="Bool"() -> ("Position:Left"=w484:i32)  [unwired: 2 in, 2 out]
                n316 = Add(x=w484, y=w482) -> (x+y=w483:i32)
                n317 = property on="new remote" class="Bool"("Position:Top"=w485, "Position:Left"=w483) -> ()  [unwired: 2 in, 2 out]
              }
            }
          }
          frame #2 {
            n318 = property class="VI"() -> ("Front Panel"=w507:refnum<vi>)  [unwired: 2 in, 2 out]
            n319 = property class="Pnl"(reference=w507, "Defer Panel Updates"=FALSE) -> ()  [unwired: 1 in, 2 out]
          }
        }
      }
      frame "ablement" {
        w522 = u8 2 items=["enabled", "disabled", "grayed"] ("disabled state")
        w523 = u8 0 items=["enabled", "disabled", "grayed"] ("disabled state")
        # "empty"
        # "empty"
        # "not selected"
        # "open directory"
        # "file"
        # "not selected"
        # "open directory"
        # "file"
        n320 = invoke on="local tree" class="Tree (strict)" method="Navigate Tree.Get Child"("Tag"="local tree") -> ("Navigate Tree:Get Child"=w515:string)  [unwired: 3 in, 3 out]
        n321 = invoke on="remote tree" class="Tree (strict)" method="Navigate Tree.Get Child"("Tag"="remote tree") -> ("Navigate Tree:Get Child"=w513:string)  [unwired: 3 in, 3 out]
        n322 = property on="local tree" class="Tree (strict)"("Active Item:Tag"="local tree") -> ("Active Item:Child-Only?"=w516:bool, "Active Item:Open?"=w518:bool)  [unwired: 2 in, 2 out]
        n323 = property on="remote tree" class="Tree (strict)"("Active Item:Tag"="remote tree") -> ("Active Item:Child-Only?"=w517:bool, "Active Item:Open?"=w521:bool)  [unwired: 2 in, 2 out]
        n324 = Empty String/Path?(string/path="local tree") -> (empty?=w525:bool)
        n325 = Empty String/Path?(string/path="remote tree") -> (empty?=w524:bool)
        n326 = Compound Arithmetic op=AND(invert w516, w518) -> (w519:bool)
        n327 = Compound Arithmetic op=AND(invert w517, w521) -> (w520:bool)
        n328 = Empty String/Path?(string/path=w515) -> (empty?=w514:bool)
        n329 = Empty String/Path?(string/path=w513) -> (empty?=w512:bool)
        n330 = stacked-sequence {
          tunnel: w519 -> [w527 w550 _ _ _ _ w580 w592 w600]
          tunnel: w525 -> [w528 w549 _ w562 _ _ w578 w591 w599]
          tunnel: w520 -> [w530 _ w554 _ _ w573 _ w589 w597]
          tunnel: w524 -> [w532 _ w553 _ w563 w569 _ w588 w596]
          tunnel: w523 -> [_ w552 w558 w561 w566 w575 w585 w594 w602]
          tunnel: w522 -> [_ w551 w557 w560 w565 w574 w584 w593 w601]
          tunnel: w517 -> [_ _ _ _ _ w571 _ _ _]
          tunnel: w516 -> [_ _ _ _ _ _ w581 _ _]
          tunnel: w514 -> [_ _ _ _ _ _ w579 _ _]
          tunnel: w512 -> [_ _ _ _ _ w572 _ _ _]
          tunnel: "local tree" -> [w529 _ _ _ _ _ _ _ _]
          tunnel: "remote tree" -> [w531 _ _ _ _ _ _ _ _]
          frame #0 {
            n331 = case shown="False" w528 {
              tunnel: w529 -> [w536 _]
              tunnel: w527 -> [w535 _]
              frame False {
                n332 = call "ClientSrv Tag to Path.vi"("tree tag"=w536) -> ("path"=w534:path)
                n333 = case shown="False" w535 {
                  tunnel: [w537 w539] -> w533
                  tunnel: w534 -> [w538 w539]
                  frame False {
                    n334 = Strip Path(path=w538) -> (stripped path=w537:path)  [unwired: 1 out]
                  }
                  frame True {
                  }
                }
                n335 = local write "local start path"(w533) -> ()
              }
              frame True {
              }
            }
            n336 = case shown="False" w532 {
              tunnel: w531 -> [w543 _]
              tunnel: w530 -> [w542 _]
              frame False {
                n337 = call "ClientSrv Tag to Path.vi"("tree tag"=w543) -> ("path"=w541:path)
                n338 = case shown="False" w542 {
                  tunnel: [w544 w546] -> w540
                  tunnel: w541 -> [w545 w546]
                  frame False {
                    n339 = Strip Path(path=w545) -> (stripped path=w544:path)  [unwired: 1 out]
                  }
                  frame True {
                  }
                }
                n340 = local write "remote start path"(w540) -> ()
              }
              frame True {
              }
            }
          }
          frame #1 {
            n341 = Compound Arithmetic op=AND(w550, invert w549) -> (w548:bool)
            n342 = Select(t=w552, s=w548, f=w551) -> (s? t:f=w547:u8)
            n343 = property on="new local" class="Bool"("Disabled"=w547) -> ()  [unwired: 2 in, 2 out]
            n344 = property on="mkdir local" class="Bool"("Disabled"=w547) -> ()  [unwired: 2 in, 2 out]
          }
          frame #2 {
            n345 = Compound Arithmetic op=AND(w554, invert w553) -> (w556:bool)
            n346 = Select(t=w558, s=w556, f=w557) -> (s? t:f=w555:u8)
            n347 = property on="new remote" class="Bool"("Disabled"=w555) -> ()  [unwired: 2 in, 2 out]
            n348 = property on="mkdir remote" class="Bool"("Disabled"=w555) -> ()  [unwired: 2 in, 2 out]
          }
          frame #3 {
            n349 = Select(t=w560, s=w562, f=w561) -> (s? t:f=w559:u8)
            n350 = property on="rename local" class="Bool"("Disabled"=w559) -> ()  [unwired: 2 in, 2 out]
          }
          frame #4 {
            n351 = Select(t=w565, s=w563, f=w566) -> (s? t:f=w564:u8)
            n352 = property on="rename remote" class="Bool"("Disabled"=w564) -> ()  [unwired: 2 in, 2 out]
          }
          frame #5 {
            n353 = And(x=w573, y=w572) -> (x .and. y?=w570:bool)
            n354 = Or(x=w571, y=w570) -> (x .or. y?=w568:bool)
            n355 = Compound Arithmetic op=AND(w568, invert w569) -> (w567:bool)
            n356 = Select(t=w575, s=w567, f=w574) -> (s? t:f=w576:u8)
            n357 = property on="delete remote" class="Bool"("Disabled"=w576) -> ()  [unwired: 2 in, 2 out]
          }
          frame #6 {
            n358 = And(x=w580, y=w579) -> (x .and. y?=w583:bool)
            n359 = Or(x=w581, y=w583) -> (x .or. y?=w582:bool)
            n360 = Compound Arithmetic op=AND(w582, invert w578) -> (w577:bool)
            n361 = Select(t=w585, s=w577, f=w584) -> (s? t:f=w586:u8)
            n362 = property on="delete local" class="Bool"("Disabled"=w586) -> ()  [unwired: 2 in, 2 out]
          }
          frame #7 {
            n363 = Compound Arithmetic op=AND(invert w592, invert w591, w589, invert w588) -> (w590:bool)
            n364 = Select(t=w594, s=w590, f=w593) -> (s? t:f=w587:u8)
            n365 = property on="upload" class="Bool"("Disabled"=w587) -> ()  [unwired: 2 in, 2 out]
          }
          frame #8 {
            n366 = Compound Arithmetic op=AND(w600, invert w599, invert w597, invert w596) -> (w598:bool)
            n367 = Select(t=w602, s=w598, f=w601) -> (s? t:f=w595:u8)
            n368 = property on="download" class="Bool"("Disabled"=w595) -> ()  [unwired: 2 in, 2 out]
          }
        }
      }
      frame "cleanup" {
        w611 = T2[] [enum."stop"] items=["empty queue", "initialize", "delayed update", "resize", "update trees", "ablement", "cleanup", "stop"]
        n369 = local read "file manipulation"() -> (w606:T1)
        n370 = invoke on="local tree" class="TreeControl (strict)" method="Edit Tree Items.Delete"("tag"="", "Delete Children"=TRUE) -> ()  [unwired: 3 in, 5 out]
        n371 = invoke on="remote tree" class="TreeControl (strict)" method="Edit Tree Items.Delete"("tag"="", "Delete Children"=TRUE) -> ()  [unwired: 3 in, 5 out]
        n372 = local write "pattern"("") -> ()
        n373 = call "obj_Library Session.vi"("method"=t_Library_Session_Methods."delist") -> ()  [unwired: 11 in, 4 out]
        n374 = call "Libary Persist Position and Controls.vi"("action"=enum16{"save", "load"}."save") -> ()  [unwired: 13 in, 2 out]
        n375 = Close Reference(reference=w606) -> ()  [unwired: 1 in, 1 out]
      }
      frame "stop" {
        n376 = invoke class="VI" method="FP.Close"() -> ()  [unwired: 3 in, 3 out]
      }
    }
  }
